vi "维持时间脚本.vi"(1 "参数":T1) -> (0 "Script":string)   [LabVIEW 2020]
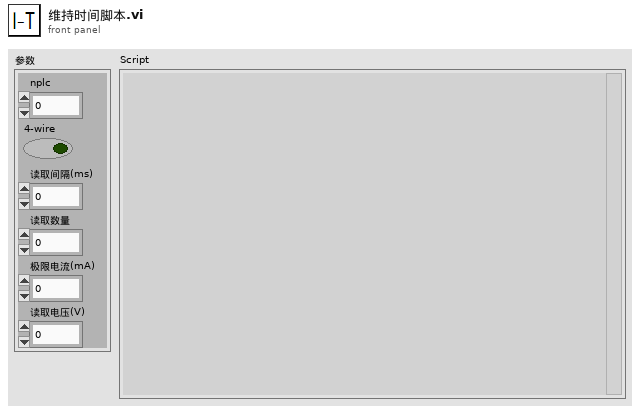
[diagram p1: front panel]
types:
  T1 = cluster{"nplc":dbl, "4-wire":bool, "读取间隔(ms)":dbl, "读取数量":dbl, "极限电流(mA)":dbl, "读取电压(V)":dbl}
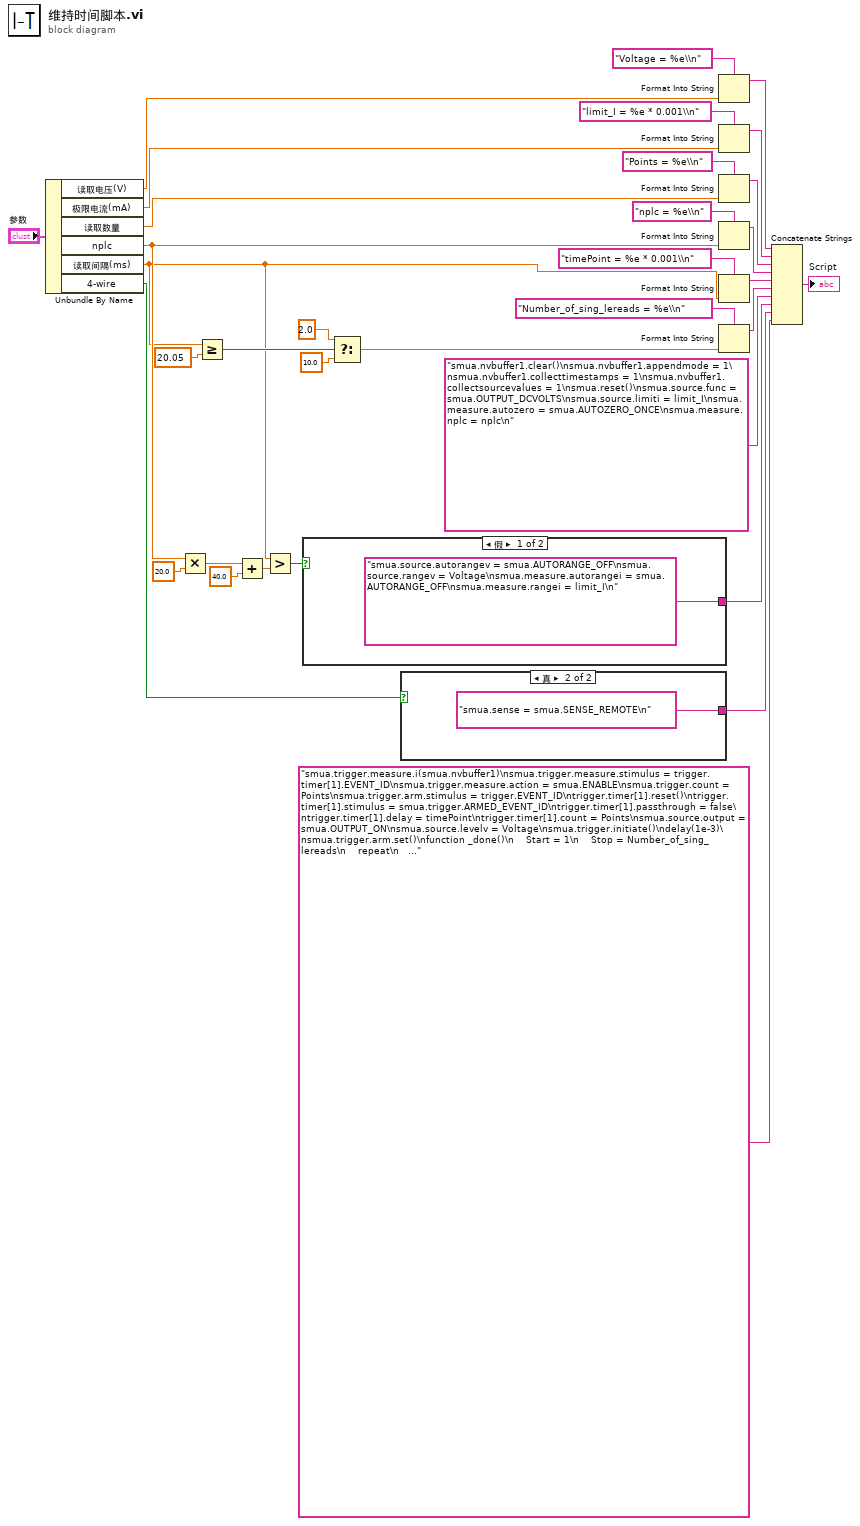
[diagram p0: block diagram]
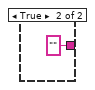
[diagram p2: hidden frame]
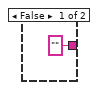
[diagram p3: hidden frame]
diagram:
  n1 = Unbundle By Name("参数") -> ("读取电压(V)"=w20:dbl, "极限电流(mA)"=w19:dbl, "读取数量"=w18:dbl, "nplc"=w9:dbl, "读取间隔(ms)"=w5:dbl, "4-wire"=w15:bool)
  n2 = Multiply(x=w9, y=20.0) -> (x*y=w7:dbl)
  n3 = Greater Or Equal?(x=w5, y=20.05) -> (x >= y?=w13:bool)
  n4 = Add(x=w7, y=40.0) -> (x+y=w4:dbl)
  n5 = Greater?(x=w5, y=w4) -> (0:w3:bool)
  n6 = case shown="假" w3 {
    tunnel: ["smua.source.autorangev = smua.AUTORANGE_OFF\nsmua.source.rangev = Voltage\nsmua.measure.autorangei = smua.AUTORANGE_OFF\nsmua.measure.rangei = limit_I\n" ""] -> w2
    frame False {
    }
    frame True {
    }
  }
  n7 = Select(t=2.0, s=w13, f=10.0) -> (s? t:f=w10:dbl)
  n8 = case shown="真" w15 {
    tunnel: ["" "smua.sense = smua.SENSE_REMOTE\n"] -> w1
    frame False {
    }
    frame True {
    }
  }
  n9 = Format Into String(format string="Voltage = %e\\n" ("格式字符串"), w20) -> (resulting string=w32:string)  [unwired: 2 in, 1 out]
  n10 = Format Into String(format string="limit_I = %e * 0.001\\n" ("格式字符串"), w19) -> (resulting string=w25:string)  [unwired: 2 in, 1 out]
  n11 = Format Into String(format string="Points = %e\\n", w18) -> (resulting string=w24:string)  [unwired: 2 in, 1 out]
  n12 = Format Into String(format string="nplc = %e\\n", w9) -> (resulting string=w23:string)  [unwired: 2 in, 1 out]
  n13 = Format Into String(format string="timePoint = %e * 0.001\\n" ("格式字符串"), w5) -> (resulting string=w22:string)  [unwired: 2 in, 1 out]
  n14 = Format Into String(format string="Number_of_sing_lereads = %e\\n" ("格式字符串"), w10) -> (resulting string=w21:string)  [unwired: 2 in, 1 out]
  n15 = Concatenate Strings(w32, w25, w24, w23, w22, w21, "smua.nvbuffer1.clear()\nsmua.nvbuffer1.appendmode = 1\nsmua.nvbuffer1.collecttimestamps = 1\nsmua.nvbuffer1.collectsourcevalues = 1\nsmua.reset()\nsmua.source.func = smua.OUTPUT_DCVOLTS\nsmua.source.limiti = limit_I\nsmua.measure.autozero = smua.AUTOZERO_ONCE\nsmua.measure.nplc = nplc\n", w2, w1, "smua.trigger.measure.i(smua.nvbuffer1)\nsmua.trigger.measure.stimulus = trigger.timer[1].EVENT_ID\nsmua.trigger.measure.action = smua.ENABLE\nsmua.trigger.count = Points\nsmua.trigger.arm.stimulus = trigger.EVENT_ID\ntrigger.timer[1].reset()\ntrigger.timer[1].stimulus = smua.trigger.ARMED_EVENT_ID\ntrigger.timer[1].passthrough = false\ntrigger.timer[1].delay = timePoint\ntrigger.timer[1].count = Points\nsmua.source.output = smua.OUTPUT_ON\nsmua.source.levelv = Voltage\nsmua.trigger.initiate()\ndelay(1e-3)\nsmua.trigger.arm.set()\nfunction _done()\n    Start = 1\n    Stop = Number_of_sing_lereads\n    repeat\n        if (bit.test(status.operation.instrument.smua.condition, 4) == false) then\n            smua.source.leveli = 0\n            smua.source.levelv = 0\n            smua.source.output = smua.OUTPUT_OFF\n            Stop = Points\n            print(\"{\" .. Stop - Start + 1 .. \"}\")\n            printbuffer(Start, Stop, smua.nvbuffer1.timestamps)\n            printbuffer(Start, Stop, smua.nvbuffer1.sourcevalues)\n            printbuffer(Start, Stop, smua.nvbuffer1)\n            print(\"{done}\")\n            return\n        elseif (smua.nvbuffer1.n > Stop) then\n            print(\"{\" .. Number_of_sing_lereads .. \"}\")\n            printbuffer(Start, Stop, smua.nvbuffer1.timestamps)\n            printbuffer(Start, Stop, smua.nvbuffer1.sourcevalues)\n            printbuffer(Start, Stop, smua.nvbuffer1)\n            Start = Start + Number_of_sing_lereads\n            Stop = Stop + Number_of_sing_lereads\n        end\n        delay(timePoint)\n    until (false)\nend\n_done()\nreset()\n") -> (→"Script":string)
